vi "Get BC.vi"(8 "error in (no error)":errorcluster, 10 "Domain":refnum<class "NI_Domain.lvclass">, 11 "BC_Evolut_2D_Numeric in":refnum<class "NI_BC_Evolut_2D_Numeric.lvclass">) -> (0 "error out":errorcluster, 2 "BC":variant, 3 "BC_Evolut_2D_Numeric out":refnum<class "NI_BC_Evolut_2D_Numeric.lvclass">)   [LabVIEW 2020, in "NI_PDE.lvlib" / "NI_BC_Evolut_2D_Numeric.lvclass"]
uses:
  <vilib>/gmath/pde.llb/BCClass/BC_Evolut_2D_Numeric/NI_BC_Evolut_2D_Numeric.lvclass
  <vilib>/gmath/pde.llb/DomainClass/NI_Domain.lvclass
  <vilib>/gmath/pde.llb/BCClass/BC_Evolut_2D_Numeric/BC Data.ctl
  <vilib>/gmath/pde.llb/Common/PDE_BC Type.ctl
  <vilib>/gmath/pde.llb/Common/PDE_BC Position 2D.ctl
  <vilib>/gmath/pde.llb/BCClass/BC_Evolut_2D_Numeric/NI_BC_Evolut_2D_Numeric.lvclass/NI_BC_Evolut_2D_Numeric.ctl
  <vilib>/gmath/NI_PDE.lvlib
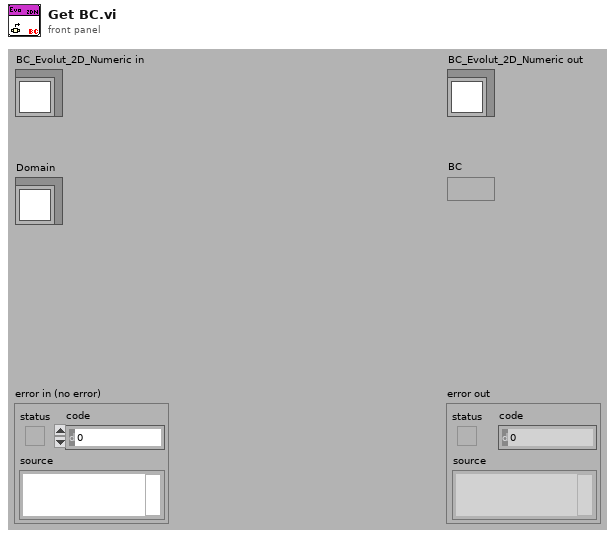
[diagram p1: front panel]
types:
  T1 = typedef "NI_PDE.lvlib/NI_BC_Evolut_2D_Numeric.lvclass/BC Data.ctl" = cluster{"type":T2, "position":T3, "G":dbl[][]}
  T2 = typedef "NI_PDE.lvlib/PDE_BC Type.ctl" = i32
  T3 = typedef "NI_PDE.lvlib/PDE_BC Position 2D.ctl" = i32
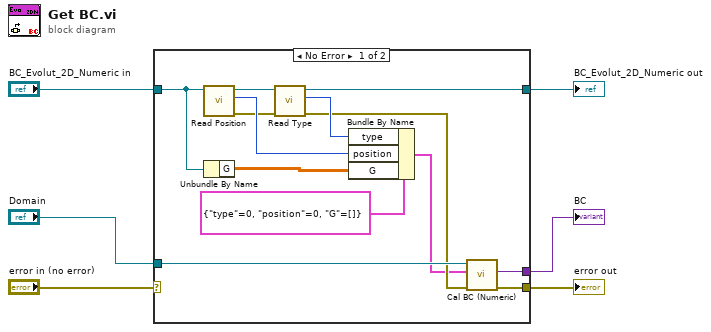
[diagram p0: block diagram]
diagram:
  n1 = case shown="No Error" "error in (no error)" {
    selector: "error in (no error)" -> [_ w20]
    tunnel: "BC_Evolut_2D_Numeric in" -> [w15 w21]
    tunnel: [w17 _] -> w4
    tunnel: [w18 w20] -> w5
    tunnel: "Domain" -> [w19 _]
    tunnel: [w13 w21] -> w3
    frame No Error {
      n2 = call-dynamic "Read Position.vi"("BC_Evolut_2D.lvclass in"=w15) -> ("error out"=w10:errorcluster, "BC position 2D"=w11:T3, "BC_Evolut_2D.lvclass out"=w14:refnum<class "NI_BC_Evolut_2D_Numeric.lvclass">)  [unwired: 1 in, 7 out]
      n3 = Unbundle By Name(w15) -> ("G"=w9:dbl[][])
      n4 = call-dynamic "Read Type.vi"("error in (no error)"=w10, "BC.lvclass in"=w14) -> ("error out"=w8:errorcluster, "BC type"=w12:T2, "BC.lvclass out"=w13:refnum<class "NI_BC_Evolut_2D_Numeric.lvclass">)  [unwired: 7 out]
      n5 = Bundle By Name(cluster=T1 {"type"=0, "position"=0, "G"=[]} ("BC data"), "type"=w12, "position"=w11, "G"=w9) -> (w7:T1)
      n6 = call-dynamic "Cal BC (Numeric).vi"("error in (no error)"=w8, "BC in"=w7, "Domain in"=w19) -> ("error out"=w18:errorcluster, "BC out"=w17:variant)  [unwired: 7 out]
    }
    frame Error {
    }
  }
  "BC" <- w4
  "error out" <- w5
  "BC_Evolut_2D_Numeric out" <- w3
